vi "solar_read MainIsMain.vi"(8 "error in (no error)":errorcluster, 11 "solar in":refnum<class "solar.lvclass">) -> (0 "error out":errorcluster, 2 "IsMain?":bool, 3 "solar out":refnum<class "solar.lvclass">)   [LabVIEW 2018, in "solar.lvclass"]
doc: "This returns true if this target is the top level main target."
uses:
  solar.lvclass
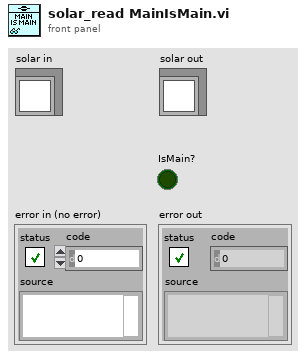
[diagram p1: front panel]
types:
  T1 = typedef "solar_ctl SOLAR Refnum.ctl" = refnum<k1>
  T2 = typedef "solar_ctl SOLAR Global.ctl" = cluster{"Targets":T3[], "AppDir":path, "solar.ini":path, "ConfigsDir":path, "CosmosDir":path, "LogsDir":path, "ExePath":path, "ExeVersion":string, "PartNum":string, "AppSetup":string, "Title":string, "Main.ini":path, "Temp.ini":path, "vSOLAR":string, "Splash.png":string, "SplashWait":i32, "SOLARUE":refnum<user-event>, "VoyagerRefnum":T4, "QTimerRefnum":T5}
  T3 = typedef "solar_ctl Target Global.ctl" = cluster{"Target":string, "Q":refnum<queue>, "UE":refnum<user-event>, "VI":refnum<vi>, "Menu":refnum<k9>, "Data":refnum<data-value>, "Attributes":variant}
  T4 = typedef "solar_voy_ctl Voyager Refnum.ctl" = refnum<k1>
  T5 = typedef "solar_qtimer_ctl Refnum.ctl" = refnum<k1>
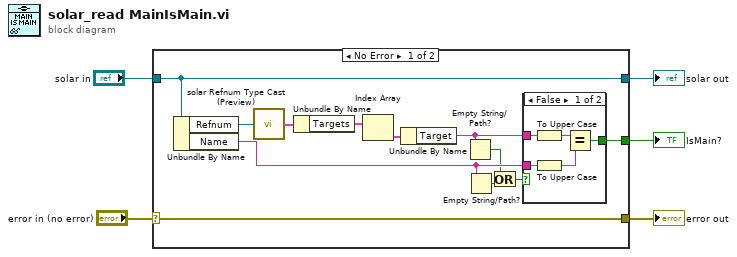
[diagram p0: block diagram]
diagram:
  n1 = case shown="No Error" "error in (no error)" {
    selector: "error in (no error)" -> [w13 w24]
    tunnel: "solar in" -> [w12 w23]
    tunnel: [w17 _] -> w4
    tunnel: [w13 w24] -> w3
    tunnel: [w12 w23] -> w1
    frame No Error {
      n2 = Unbundle By Name(w12) -> ("Refnum"=w11:T1, "Name"=w16:string)
      n3 = call "solar Refnum Type Cast (Preview).vi"("Refnum"=w11) -> ("SOLAR"=w10:T2)  [unwired: 8 in]
      n4 = Unbundle By Name(w10) -> ("Targets"=w9:T3[])
      n5 = Index Array(array=w9) -> (element=w8:T3)  [unwired: 1 in]
      n6 = Unbundle By Name(w8) -> ("Target"=w6:string)
      n7 = Empty String/Path?(string/path=w6) -> (empty?=w7:bool)
      n8 = Empty String/Path?(string/path=w16) -> (empty?=w15:bool)
      n9 = Or(x=w7, y=w15) -> (x .or. y?=w14:bool)
      n10 = case shown="False" w14 {
        tunnel: [w20 _] -> w17
        tunnel: w16 -> [w19 _]
        tunnel: w6 -> [w18 _]
        frame False {
          n11 = To Upper Case(1:w18) -> (0:w22:string)
          n12 = To Upper Case(1:w19) -> (0:w21:string)
          n13 = Equal?(x=w22, y=w21) -> (x = y?=w20:bool)
        }
        frame True {
        }
      }
    }
    frame Error {
    }
  }
  "error out" <- w3
  "solar out" <- w1
  "IsMain?" <- w4
